vi "Dequeue Message.vi"(8 "error in (no error)":errorcluster, 11 "Message Queue":refnum<queue>) -> (0 "error out":errorcluster, 1 "Message Data":variant, 2 "developer_test sequence":T1 caption="Enum", 3 "dup Message Queue":refnum<queue>)   [LabVIEW 2021, in "RMU Message Queue.lvlib"]
doc: "This VI pulls messages off the Message Queue."
uses:
  RMU Message Queue.lvlib
  Message Cluster.ctl
  controls/developer_test sequence.ctl
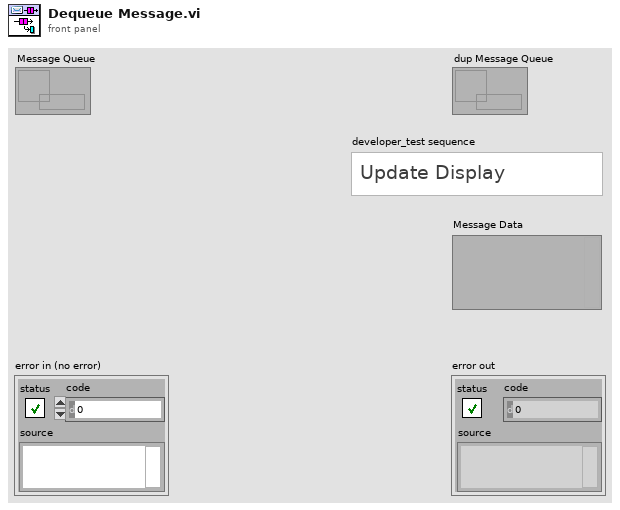
[diagram p1: front panel]
types:
  T1 = typedef "developer_test sequence.ctl" = enum16{"Update Display", "User Login", "Initialise", "Init Devices", "Idle State", "Check All", "UnCheck All", "test steup", "Abort", "Start Display Board Auto Testing", "Scan Barcode", "Check 5V Short", "Power on DUT(5V Power Supply)", "Programming", "current firmware", "RS485 Communication", "Load Cell High", "Load Cell Mid", "Load Cell Low", "Stop Display Board Auto Testing", "All Pass", "Fail", "Report", "Error", "Confirm Quit", "Exit"}
  T2 = typedef "RMU Message Queue.lvlib/Message Cluster.ctl" = cluster{"test sequence":T1, "Message Data":variant}
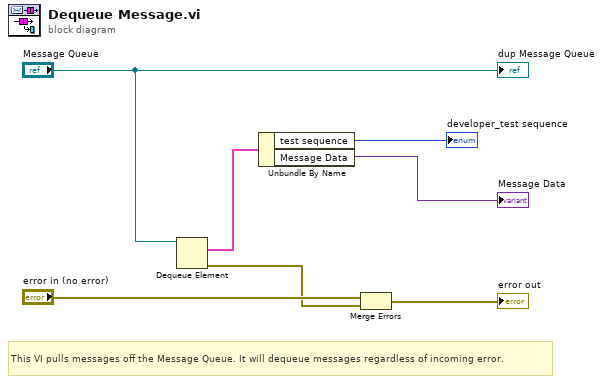
[diagram p0: block diagram]
diagram:
  # "This VI pulls messages off the Message Queue. It will dequeue messages regardless of incoming error."
  n1 = Dequeue Element(queue="Message Queue") -> (element=w5:T2, error out=w2:errorcluster)  [unwired: 2 in, 2 out]
  n2 = Unbundle By Name(w5) -> ("test sequence"=→"developer_test sequence":T1, "Message Data"=→"Message Data":variant)
  n3 = Merge Errors("error in (no error)", w2) -> (→"error out":errorcluster)
  "dup Message Queue" <- "Message Queue"
